vi "Get Headers.vi"(6 "timeout (10000)":i32=10000, 8 "error in (no error)":errorcluster, 11 "URL":string) -> (0 "error out":errorcluster, 1 "Response String":string, 2 "Headers":map{string, string}(c390), 3 "Reponse Code":i32, 5 "Version":string, 7 "Protocol":string)   [LabVIEW 2020, in "binary_installation_tools.lvlib"]
uses:
  binary_installation_tools.lvlib
  <vilib>/httpClient/LabVIEWHTTPClient.lvlib
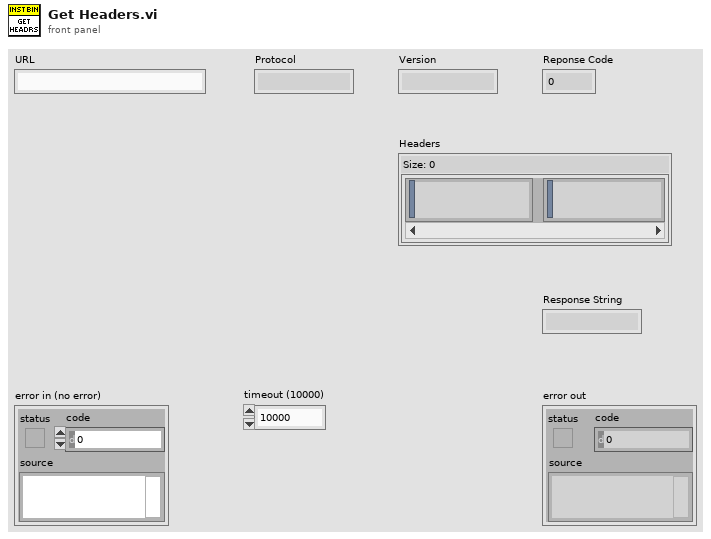
[diagram p1: front panel]
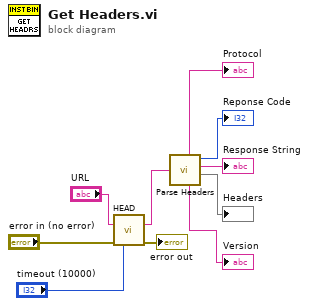
[diagram p0: block diagram]
diagram:
  n1 = call <vilib>:"HEAD.vi"("url"="URL", "error in (no error)"="error in (no error)", "timeout (10000)"="timeout (10000)") -> ("headers"=w9:string, "error out"=→"error out":errorcluster)  [unwired: 10 in, 1 out]
  n2 = call "Parse Headers.vi"("Headers"=w9) -> ("Version"=→"Version":string, "Map"=→"Headers":map{string, string}, "Response"=→"Response String":string, "Protocol"=→"Protocol":string, "Response Code"=→"Reponse Code":i32)  [unwired: 3 in]
